vi "Destroy.vi"(8 "error in (no error)":errorcluster, 9 "Test Mode":bool, 11 "Sift Client in":refnum<class "Sift Client.lvclass">) -> (0 "error out":errorcluster, 3 "Sift Client out":refnum<class "Sift Client.lvclass">)   [LabVIEW 2024, in "Sift Client.lvlib" / "Sift Client.lvclass"]
doc: "Releases resources used by the Sift Client."
uses:
  Sift Client.lvclass
  Sift Client.lvclass/Sift Client.ctl
  <vilib>/addons/_JKI.lib/REST Client/classes/REST Client/REST Client.lvclass
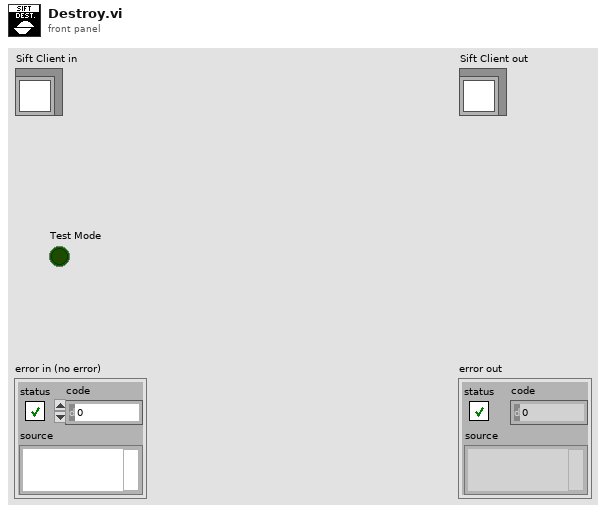
[diagram p1: front panel]
types:
  T1 = typedef "Sift Client.lvlib/Data Queue.ctl" = cluster{"String Queue":refnum<queue>, "Double Queue":refnum<queue>, "Float Queue":refnum<queue>, "Int64 Queue":refnum<queue>, "Bool Queue":refnum<queue>, "Int32 Queue":refnum<queue>, "Uint64 Queue":refnum<queue>, "Uint32 Queue":refnum<queue>, "Enum Queue":refnum<queue>, "Bitfield Queue":refnum<queue>}
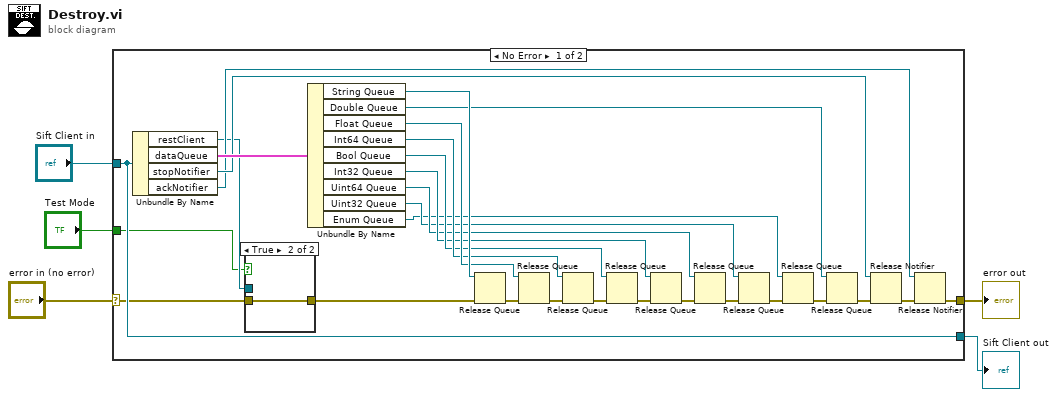
[diagram p0: block diagram]
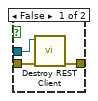
[diagram p2: hidden frame]
diagram:
  n1 = case shown="No Error" "error in (no error)" {
    selector: "error in (no error)" -> [w9 w39]
    tunnel: [w10 w39] -> w4
    tunnel: [w33 w38] -> w2
    tunnel: "Sift Client in" -> [w33 w38]
    tunnel: "Test Mode" -> [w6 _]
    frame No Error {
      n2 = Unbundle By Name(w33) -> ("restClient"=w8:refnum<class "REST Client.lvclass">, "dataQueue"=w32:T1, "stopNotifier"=w14:refnum<notifier>, "ackNotifier"=w13:refnum<notifier>)
      n3 = case shown="True" w6 {
        tunnel: w9 -> [w36 w37]
        tunnel: w8 -> [w35 _]
        tunnel: [w34 w37] -> w7
        frame False {
          n4 = call-dynamic "Destroy REST Client.vi"("error in (no error)"=w36, "REST Client in"=w35) -> ("error out"=w34:errorcluster)  [unwired: 9 in]
        }
        frame True {
        }
      }
      n5 = Unbundle By Name(w32) -> ("String Queue"=w31:refnum<queue>, "Double Queue"=w30:refnum<queue>, "Float Queue"=w29:refnum<queue>, "Int64 Queue"=w28:refnum<queue>, "Bool Queue"=w27:refnum<queue>, "Int32 Queue"=w26:refnum<queue>, "Uint64 Queue"=w25:refnum<queue>, "Uint32 Queue"=w24:refnum<queue>, "Enum Queue"=w23:refnum<queue>)
      n6 = Release Queue(queue=w31, error in (no error)=w7) -> (error out=w22:errorcluster)  [unwired: 1 in, 2 out]
      n7 = Release Queue(queue=w29, error in (no error)=w22) -> (error out=w21:errorcluster)  [unwired: 1 in, 2 out]
      n8 = Release Queue(queue=w28, error in (no error)=w21) -> (error out=w20:errorcluster)  [unwired: 1 in, 2 out]
      n9 = Release Queue(queue=w27, error in (no error)=w20) -> (error out=w19:errorcluster)  [unwired: 1 in, 2 out]
      n10 = Release Queue(queue=w26, error in (no error)=w19) -> (error out=w18:errorcluster)  [unwired: 1 in, 2 out]
      n11 = Release Queue(queue=w25, error in (no error)=w18) -> (error out=w17:errorcluster)  [unwired: 1 in, 2 out]
      n12 = Release Queue(queue=w24, error in (no error)=w17) -> (error out=w16:errorcluster)  [unwired: 1 in, 2 out]
      n13 = Release Queue(queue=w23, error in (no error)=w16) -> (error out=w15:errorcluster)  [unwired: 1 in, 2 out]
      n14 = Release Queue(queue=w30, error in (no error)=w15) -> (error out=w12:errorcluster)  [unwired: 1 in, 2 out]
      n15 = Release Notifier(notifier=w14, error in (no error)=w12) -> (error out=w11:errorcluster)  [unwired: 1 in, 2 out]
      n16 = Release Notifier(notifier=w13, error in (no error)=w11) -> (error out=w10:errorcluster)  [unwired: 1 in, 2 out]
    }
    frame Error {
    }
  }
  "error out" <- w4
  "Sift Client out" <- w2
